vi "Test Report is Closed on Test End.vi"(8 "error in (no error)":errorcluster, 11 "XML Report Test in":refnum<class "Report Generator Test.lvclass">) -> (0 "error out":errorcluster, 3 "XML Report Test out":refnum<class "Report Generator Test.lvclass">)   [LabVIEW 2020, in "Report Generator Test.lvclass"]
uses:
  Report Generator Test.lvclass
  C:/Program Files (x86)/National Instruments/LabVIEW 2020/vi.lib/Astemes/LUnit/Core/LUnit Test Case/Test Case.lvclass
  <vilib>/Astemes/LUnit/Core/LUnit Test Case/Test Case.lvclass/Test Case.ctl
  <vilib>/Astemes/LUnit/Core/LUnit Test Case/Private/Append Pass Result.vi
  <vilib>/Astemes/LUnit/Core/LUnit Test Case/Private/Append Fail Result.vi
  <vilib>/Astemes/LUnit/Core/LUnit Test Case/Private/Run In UI.vi
  <vilib>/Utility/error.llb/Clear Errors.vi
  Test Doubles/Mock Report/Mock Report.lvclass
  <vilib>/Astemes/LUnit/Core/LUnit Test Case/Test Case.lvclass
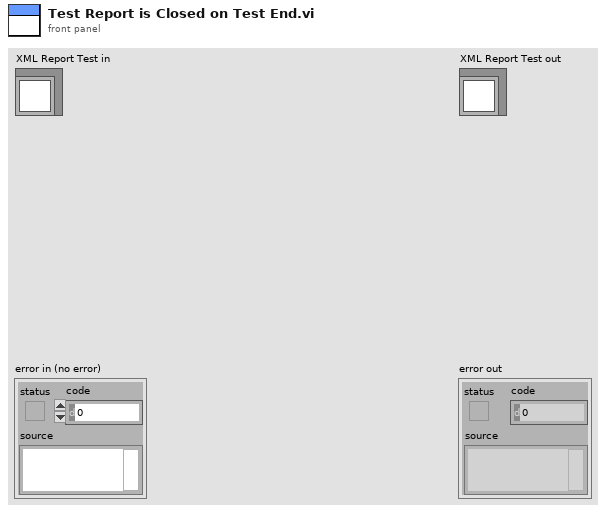
[diagram p1: front panel]
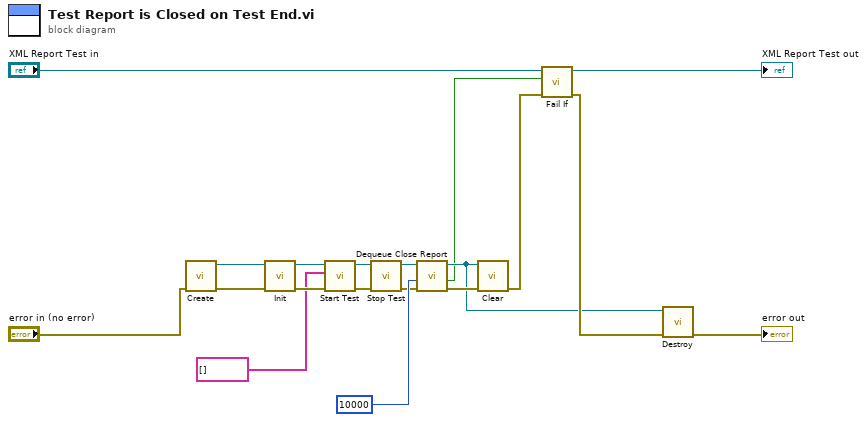
[diagram p0: block diagram]
diagram:
  n1 = call "Create.vi"("error in (no error)"="error in (no error)") -> ("error out"=w9:errorcluster, "Mock Report Out"=w11:refnum<class "Mock Report.lvclass">)  [unwired: 9 in]
  n2 = call-dynamic "Init.vi"("error in (no error)"=w9, "Mock Report In"=w11) -> ("error out"=w15:errorcluster, "Mock Report Out"=w16:refnum<class "Mock Report.lvclass">)  [unwired: 8 in]
  n3 = call-dynamic "Start Test.vi"("error in (no error)"=w15, "Tests"=string[] [], "XML Report in"=w16) -> ("error out"=w14:errorcluster, "XML Report out"=w2:refnum<class "Mock Report.lvclass">)  [unwired: 7 in]
  n4 = call-dynamic "Stop Test.vi"("error in (no error)"=w14, "XML Report in"=w2) -> ("error out"=w3:errorcluster, "XML Report out"=w1:refnum<class "Mock Report.lvclass">)  [unwired: 8 in]
  n5 = call "Dequeue Close Report.vi"("error in (no error)"=w3, "timeout in ms (0)"=10000, "Mock Report In"=w1) -> ("error out"=w13:errorcluster, "timed out?"=w4:bool, "Mock Report Out"=w7:refnum<class "Mock Report.lvclass">)  [unwired: 6 in]
  n6 = call-dynamic "Clear.vi"("error in (no error)"=w13, "XML Report in"=w7) -> ("error out"=w12:errorcluster)  [unwired: 9 in]
  n7 = call <vilib>:"Fail If.vi"("error in (no error)"=w12, "Fail?"=w4, "LUnit Test Case In"="XML Report Test in") -> ("error out"=w17:errorcluster, "LUnit Test Case Out"=→"XML Report Test out":refnum<class "Report Generator Test.lvclass">)  [unwired: 7 in]
  n8 = call "Destroy.vi"("error in (no error)"=w17, "Mock Report In"=w7) -> ("error out"=→"error out":errorcluster)  [unwired: 9 in]
